vi "URAPI_WriteDigitalOut.vi"(0 "Variable In":string, 3 "URAPI Script":T1={"Script"="", "Whiles"=[], "Ifs"=[], "Supress Err"=TRUE, "Errors"=""}, 4 "Channel":string) -> (2 "Variable Out":string, 5 "URAPI Script":T1={"Script"="", "Whiles"=[], "Ifs"=[], "Supress Err"=TRUE, "Errors"=""})   [LabVIEW 2014]
doc: "Writes the value of \"Variable In\" to the specified digital \"Channel\"."
uses:
  <userlib>/botspeak/VIs/Direct/URAPI_Control.ctl
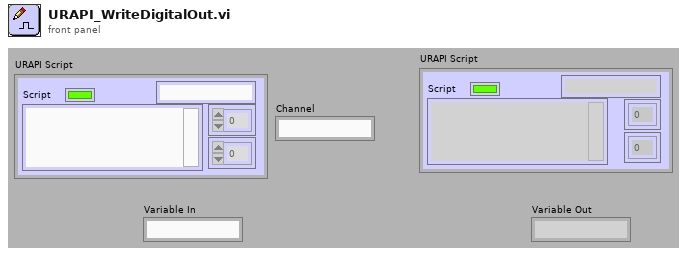
[diagram p1: front panel]
types:
  T1 = typedef "URAPI_Control.ctl" = cluster{"Script":string, "Whiles":u8[], "Ifs":u8[], "Supress Err":bool, "Errors":string}
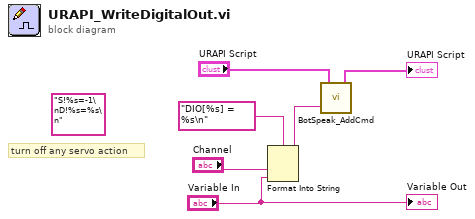
[diagram p0: block diagram]
diagram:
  (unwired) "S!%s=-1\nD!%s=%s\n" ("string")
  # "turn off any servo action"
  n1 = Format Into String(format string="DIO[%s] = %s\n" ("string"), "Channel", "Variable In") -> (resulting string=w1:string)  [unwired: 2 in, 1 out]
  n2 = call <userlib>:"BotSpeak_AddCmd.vi"("String"=w1, "URAPI Script"="URAPI Script") -> ("URAPI Script out"=→"URAPI Script":T1)  [unwired: 1 in]
  "Variable Out" <- "Variable In"
